vi "Hypotenuse_Control.vi"(9 "Deadband":dbl=0.75 format="%#_13g", 10 "Limit_Axis":dbl, 11 "Main_Axis":dbl) -> (3 "Axis_Adj":dbl)   [LabVIEW 2013]
panel:
  # "Hypotenuse Control"
  # "This subsystem finds the hypotenuse.  A deadband is then created on the limit axis. \n This was done to allow less percise modjulation of the joystikcs"
  # "Inputs"
  # "Tunning"
  # "Outputs"
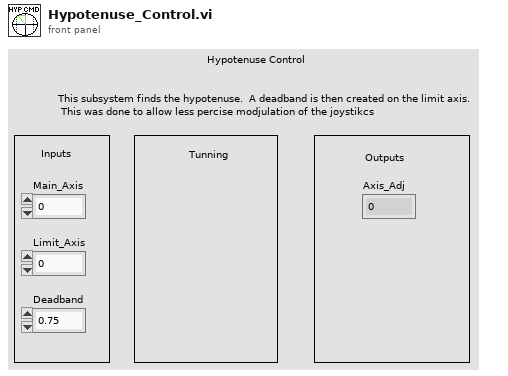
[diagram p1: front panel]
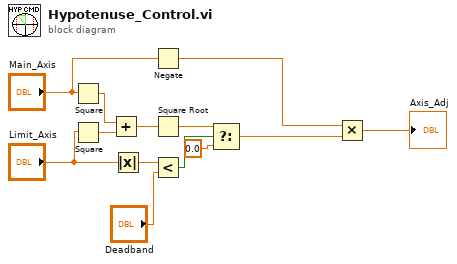
[diagram p0: block diagram]
diagram:
  n1 = Square(x="Main_Axis") -> (x^2=w12:dbl)
  n2 = Square(x="Limit_Axis") -> (x^2=w5:dbl)
  n3 = Add(x=w12, y=w5) -> (x+y=w6:dbl)
  n4 = Absolute Value(x="Limit_Axis") -> (abs(x)=w10:dbl)
  n5 = Negate(x="Main_Axis") -> (-x=w1:dbl)
  n6 = Square Root(x=w6) -> (sqrt(x)=w8:dbl)
  n7 = Less?(x=w10, y="Deadband") -> (x < y?=w13:bool)
  n8 = Select(t=w8, s=w13, f=0.0) -> (s? t:f=w4:dbl)
  n9 = Multiply(x=w1, y=w4) -> (x*y=→"Axis_Adj":dbl)
